vi "Check Spawn.vi"(9 "UID":string, 10 "Actor":refnum<class "Actor.lvclass">) -> (2 "Error":errorcluster)   [LabVIEW 2025, in "jettl.lvlib"]
uses:
  jettl.lvlib
  Actor/Actor.lvclass
  Error/Error.lvlib
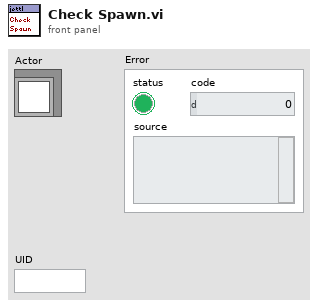
[diagram p1: front panel]
types:
  T1 = typedef "jettl.lvlib/Child UIDs.ctl" = set{string}
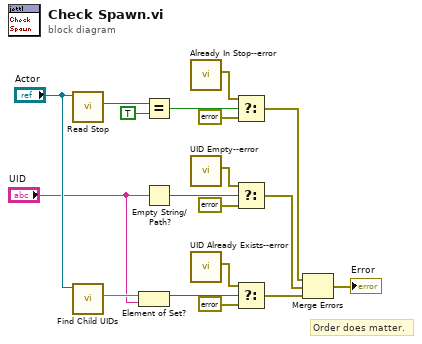
[diagram p0: block diagram]
diagram:
  # "Order does matter."
  n1 = call-dynamic "Read Stop.vi"("Actor in"="Actor") -> ("Stop"=w16:bool)  [unwired: 10 in]
  n2 = call-dynamic "Find Child UIDs.vi"("Actor in"="Actor") -> ("Child UIDs"=w18:T1)  [unwired: 10 in]
  n3 = Element of Set?(10:"UID", 11:w18) -> (3:w7:bool)
  n4 = Equal?(x=w16, y=TRUE) -> (x = y?=w14:bool)
  n5 = Empty String/Path?(string/path="UID") -> (empty?=w9:bool)
  n6 = call "Already In Stop--error.vi"() -> ("Error"=w13:errorcluster)  [unwired: 11 in]
  n7 = call "UID Empty--error.vi"() -> ("Error"=w10:errorcluster)  [unwired: 11 in]
  n8 = call "UID Already Exists--error.vi"() -> ("Error"=w11:errorcluster)  [unwired: 11 in]
  n9 = Select(t=w13, s=w14, f=errorcluster {"status"=FALSE, "code"=0, "source"=""}) -> (s? t:f=w6:errorcluster)
  n10 = Select(t=w10, s=w9, f=errorcluster {"status"=FALSE, "code"=0, "source"=""}) -> (s? t:f=w2:errorcluster)
  n11 = Select(t=w11, s=w7, f=errorcluster {"status"=FALSE, "code"=0, "source"=""}) -> (s? t:f=w1:errorcluster)
  n12 = Merge Errors(w6, w2, w1) -> (→"Error":errorcluster)
